vi "meth.GetOutputReader.vi"(0 "class.GLue in":refnum<class "class.GLue.lvclass">, 11 "error in":errorcluster) -> (4 "class.GLue out":refnum<class "class.GLue.lvclass">, 8 "ReaderContext":T1, 15 "error out":errorcluster)   [LabVIEW 2014, in "GLue.lvlib" / "class.GLue.lvclass"]
uses:
  class.GLue.lvclass
  class.GLue.lvclass/class.GLue.ctl
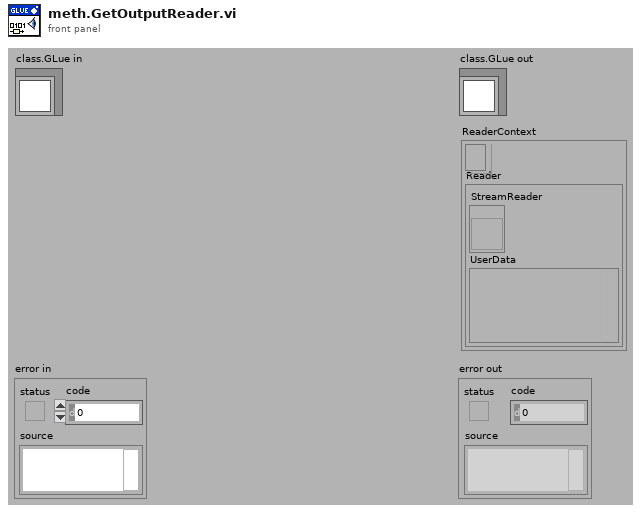
[diagram p1: front panel]
types:
  T1 = cluster{"EventRef":refnum<event-registration>, "Reader":cluster{"StreamReader":refnum<vi>, "UserData":variant}}
  T2 = cluster{"StreamReader":refnum<vi>, "UserData":variant}
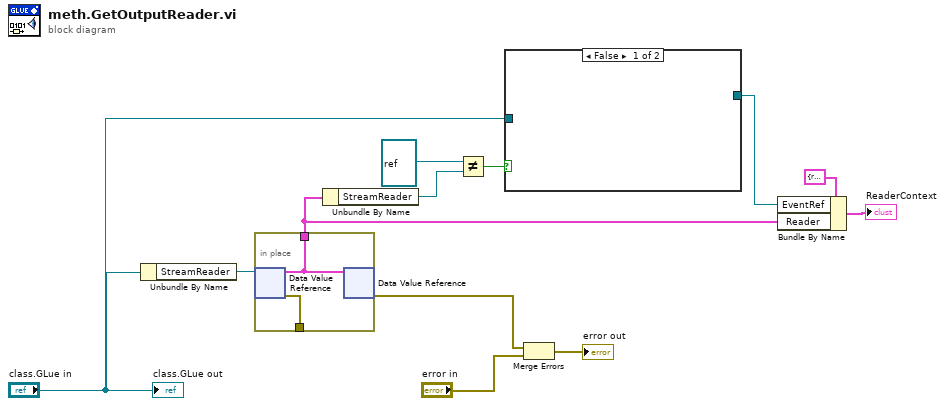
[diagram p0: block diagram]
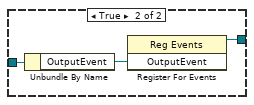
[diagram p2: hidden frame]
diagram:
  n1 = Unbundle By Name("class.GLue in") -> ("StreamReader"=w12:refnum<data-value>)
  n2 = in-place {
    in-place-border: [w14] -> _
    in-place-border: [w13] -> w3
    n3 = in-place-dvr #1(w12) -> (w13:T2, w14:errorcluster)
    n4 = in-place-dvr #1(w13) -> (w11:errorcluster)  [unwired: 1 out]
  }
  n5 = Unbundle By Name(w3) -> ("StreamReader"=w4:refnum<vi>)
  n6 = Not Equal?(x=refnum<vi> refnum ("StreamReader"), y=w4) -> (x != y?=w7:bool)
  n7 = case shown="False" w7 {
    tunnel: "class.GLue in" -> [_ w16]
    tunnel: [_ w15] -> w5
    frame False {
    }
    frame True {
      n8 = Unbundle By Name(w16) -> ("OutputEvent"=w17:refnum<user-event>)
      n9 = register-events(w17) -> (reference out=w15:refnum<event-registration>)  [unwired: 2 in, 1 out]
    }
  }
  n10 = Merge Errors(w11, "error in") -> (→"error out":errorcluster)
  n11 = Bundle By Name(cluster=T1 {"EventRef"=refnum, "Reader"={"StreamReader"=refnum, "UserData"=variant}}, "EventRef"=w5, "Reader"=w3) -> (→"ReaderContext":T1)
  "class.GLue out" <- "class.GLue in"
